vi "Create Measurement Enable Array for a part.vi"(9 "Measurement Names Array":string[](array[string]), 10 "Part Name":string, 11 "AllPartInfoArray":T1) -> (3 "Measurement Enable Array":bool[](array[boolean]))   [LabVIEW 2019, in "DataLogger.lvclass"]
uses:
  DataLogger.lvclass
  Common/Controls/AllPartInfo.ctl
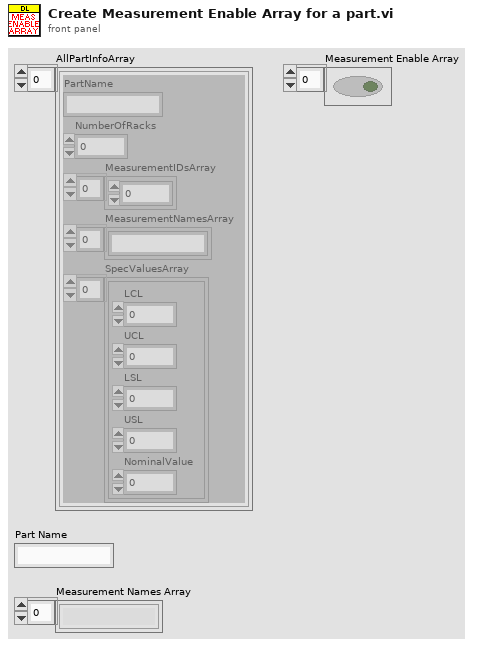
[diagram p1: front panel]
types:
  T1 = typedef "AllPartInfo.ctl" = cluster{"PartName":string, "NumberOfRacks":u8, "MeasurementIDsArray":u16[], "MeasurementNamesArray":string[], "SpecValuesArray":cluster{"LCL":dbl, "UCL":dbl, "LSL":dbl, "USL":dbl, "NominalValue":dbl}[]}[]
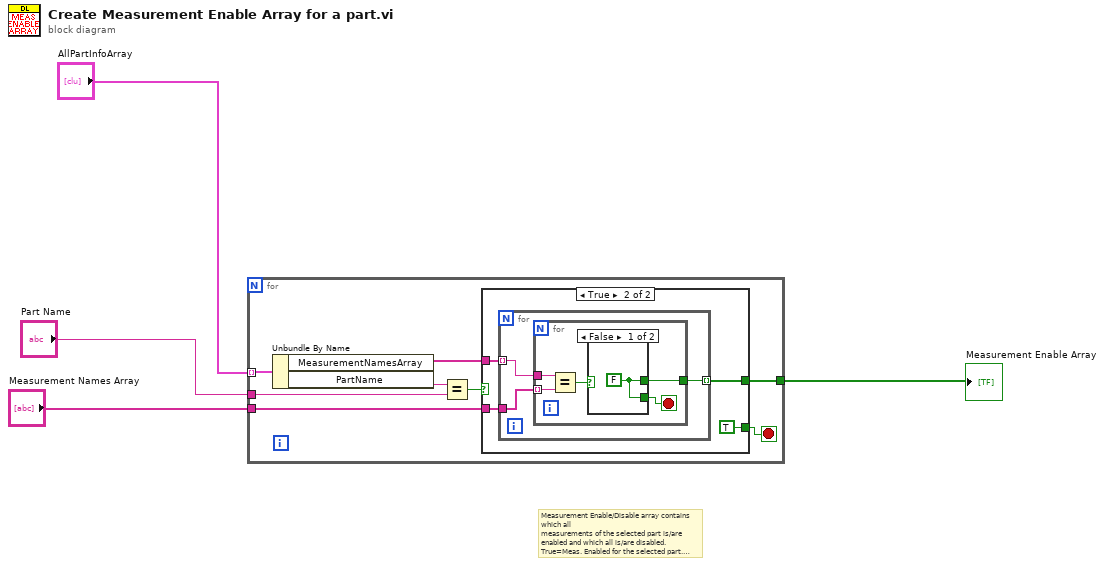
[diagram p0: block diagram]
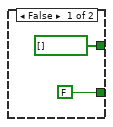
[diagram p2: hidden frame]
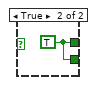
[diagram p3: hidden frame]
diagram:
  # "Measurement Enable/Disable array contains which all\nmeasurements of the selected part is/are enabled and which all is/are disabled.\nTrue=Meas. Enabled for the selected part.\nFalse=Meas. Disabled for the selected part."
  n1 = for {
    tunnel: "AllPartInfoArray" -> [w12] mode=indexing
    tunnel: "Part Name" -> [w10]
    tunnel: "Measurement Names Array" -> [w6]
    tunnel: [w5] -> w1
    stop <- w7 stop-if-true
    n2 = Unbundle By Name(w12) -> ("MeasurementNamesArray"=w8:string[], "PartName"=w11:string)
    n3 = Equal?(x=w11, y=w10) -> (x = y?=w9:bool)
    n4 = case shown="True" w9 {
      tunnel: w8 -> [_ w17]
      tunnel: [FALSE TRUE] -> w7
      tunnel: w6 -> [_ w16]
      tunnel: [bool[] [] w15] -> w5
      frame False {
      }
      frame True {
        n5 = for {
          tunnel: w17 -> [w20] mode=indexing
          tunnel: w16 -> [w21]
          tunnel: [w19] -> w15 mode=indexing
          n6 = for {
            tunnel: w21 -> [w26] mode=indexing
            tunnel: w20 -> [w25]
            tunnel: [w23] -> w19
            stop <- w22 stop-if-true
            n7 = Equal?(x=w25, y=w26) -> (x = y?=w24:bool)
            n8 = case shown="False" w24 {
              tunnel: [w27 w28] -> w23
              tunnel: [w27 w28] -> w22
              frame False {
                w27 = FALSE
              }
              frame True {
                w28 = TRUE
              }
            }
          }
        }
      }
    }
  }
  "Measurement Enable Array" <- w1
